vi "CS_Read_Config.vi"(4 "error in (no error)":errorcluster, 7 "Config refnum":T1) -> (0 "error out":errorcluster, 2 "All Found?":bool, 3 "refnum out":T1)   [LabVIEW 2015]
uses:
  <vilib>/Utility/config.llb/Config Data RefNum.ctl
  <vilib>/Utility/config.llb/Read Key (Double).vi
  GSP_Wavelength_Global.vi
  <vilib>/Utility/config.llb/NI_LVConfig.lvlib
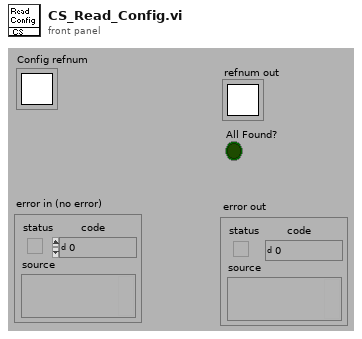
[diagram p1: front panel]
types:
  T1 = typedef "NI_LVConfig.lvlib/Config Data RefNum.ctl" = refnum<k1>
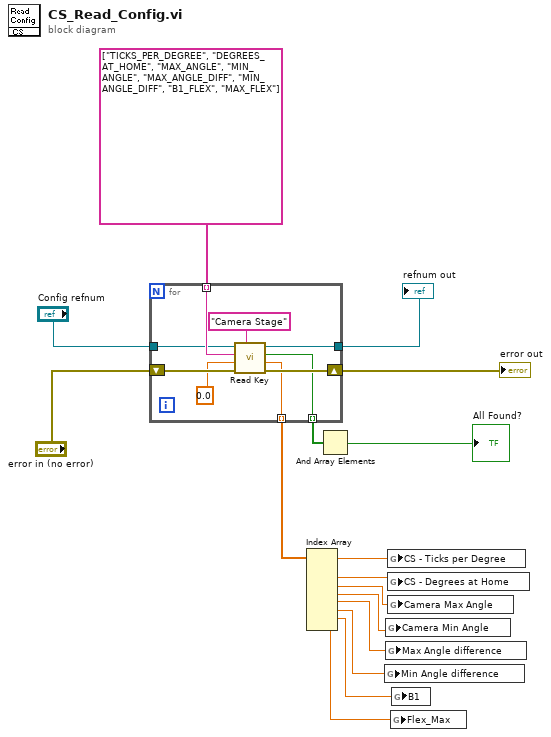
[diagram p0: block diagram]
diagram:
  n1 = for {
    shift-right: [w23] -> w16
    shift-left: "error in (no error)" -> [w25]
    tunnel: [w22] -> w15
    tunnel: string[] ["TICKS_PER_DEGREE", "DEGREES_AT_HOME", "MAX_ANGLE", "MIN_ANGLE", "MAX_ANGLE_DIFF", "MIN_ANGLE_DIFF", "B1_FLEX", "MAX_FLEX"] -> [w21] mode=indexing
    tunnel: [w20] -> w14 mode=indexing
    tunnel: [w18] -> w13 mode=indexing
    tunnel: "Config refnum" -> [w17]
    n2 = call-poly <vilib>:"Read Key.vi"("section"="Camera Stage", "error in (no error)"=w25, "default value"=0.0, "key"=w21, "refnum"=w17) -> ("error out"=w23:errorcluster, "value"=w18:dbl, "found?"=w20:bool, "refnum out"=w22:T1)  [unwired: 3 in]
  }
  "error out" <- w16
  "refnum out" <- w15
  n3 = Index Array(array=w13) -> (element #1=w8:dbl, element #2=w7:dbl, element #3=w6:dbl, element #4=w5:dbl, element #5=w4:dbl, element #6=w3:dbl, element #7=w2:dbl, element #8=w1:dbl)  [unwired: 8 in]
  n4 = And Array Elements(Boolean array=w14) -> (logical AND=→"All Found?":bool)
  n5 = global write "GSP_Wavelength_Global.vi" "Min Angle difference"(w3) -> ()
  n6 = global write "GSP_Wavelength_Global.vi" "Camera Min Angle"(w5) -> ()
  n7 = global write "GSP_Wavelength_Global.vi" "Max Angle difference"(w4) -> ()
  n8 = global write "GSP_Wavelength_Global.vi" "CS - Ticks per Degree"(w8) -> ()
  n9 = global write "GSP_Wavelength_Global.vi" "CS - Degrees at Home"(w7) -> ()
  n10 = global write "GSP_Wavelength_Global.vi" "Camera Max Angle"(w6) -> ()
  n11 = global write "GSP_Wavelength_Global.vi" "Flex_Max"(w1) -> ()
  n12 = global write "GSP_Wavelength_Global.vi" "B1"(w2) -> ()
